vi "Pressure Control StationE.vi"(8 "error in (no error)":errorcluster, 11 "Pressure Controls":bool[](array[boolean])=[FALSE, FALSE, FALSE, FALSE]) -> (0 "error out":errorcluster, 3 "Output status of pressure lines":bool[](array[boolean]))   [LabVIEW 2011]
uses:
  <vilib>/DAQmx/write.llb/DAQmx Write (Digital 1D Bool 1Chan 1Samp).vi
  <vilib>/DAQmx/create/channels.llb/DAQmx Create Channel (DO-Digital Output).vi
  <vilib>/DAQmx/miscellaneous.llb/DAQmx Fill In Error Info.vi
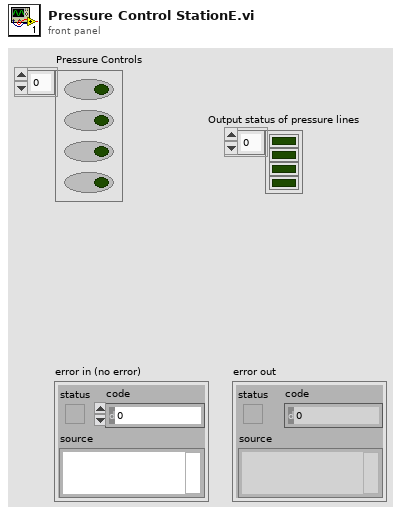
[diagram p1: front panel]
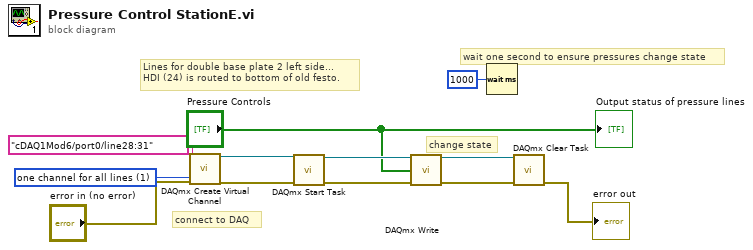
[diagram p0: block diagram]
diagram:
  w12 = 1 items=["one channel for each line", "one channel for all lines"] ("line grouping")
  # "Lines for double base plate 2 left side...\nHDI (24) is routed to bottom of old festo."
  # "change state"
  # "connect to DAQ"
  # "wait one second to ensure pressures change state"
  n1 = call-poly <vilib>:"DAQmx Create Virtual Channel.vi"("lines"=tag "cDAQ1Mod6/port0/line28:31", "line grouping"=w12, "error in"="error in (no error)") -> ("task out"=w10:refnum<k21>, "error out"=w9:errorcluster)  [unwired: 2 in, 9 out]
  n2 = call <vilib>:"DAQmx Start Task.vi"("task/channels in"=w10, "error in"=w9) -> ("task out"=w8:refnum<k21>, "error out"=w7:errorcluster)  [unwired: 12 out]
  n3 = call-poly <vilib>:"DAQmx Write.vi"("task/channels in"=w8, "data"="Pressure Controls", "error in"=w7) -> ("task out"=w6:refnum<k21>, "error out"=w5:errorcluster)  [unwired: 1 in, 10 out]
  n4 = Wait (ms)(milliseconds to wait=u32 1000) -> ()  [unwired: 1 out]
  n5 = call <vilib>:"DAQmx Clear Task.vi"("task in"=w6, "error in"=w5) -> ("error out"=→"error out":errorcluster)  [unwired: 13 out]
  "Output status of pressure lines" <- "Pressure Controls"
